vi "PRACTICA 2.vi"() -> ()   [LabVIEW 2017]
panel:
  in  "stop":bool
  in  "Knob 2":dbl(knob) scale=0.0..10.0
  in  "Knob":dbl(knob) scale=0.0..10.0
  out "RESULTADO":dbl
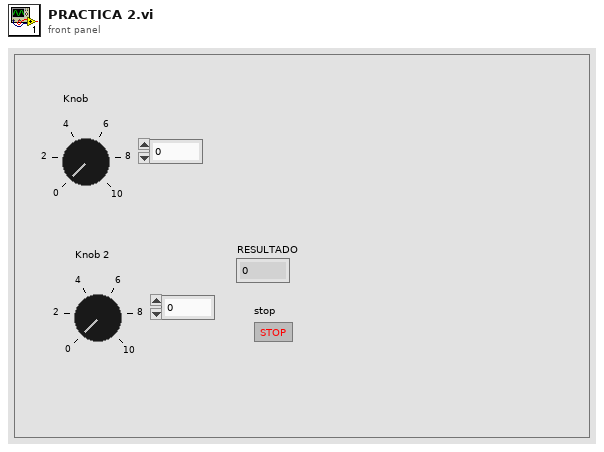
[diagram p1: front panel]
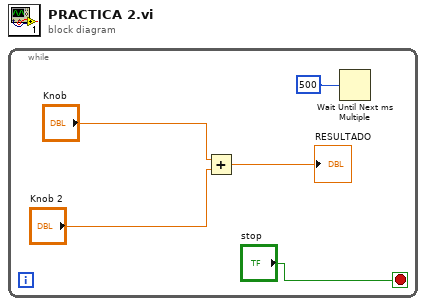
[diagram p0: block diagram]
diagram:
  n1 = while {
    stop <- "stop" stop-if-true
    n2 = Add(x="Knob", y="Knob 2") -> (x+y=→"RESULTADO":dbl)
    n3 = Wait Until Next ms Multiple(millisecond multiple=u32 500 ("millisecond timer value")) -> ()  [unwired: 1 out]
  }
